vi "FMA1600A Add Units.vi"(0 "Meter Bank 2":T1, 1 "Meter Bank 1":T1, 5 "Meter Bank 3":T1, 7 "Measurement Units 1":T3, 9 "Measurement Units 2":T3, 12 "Measurement Units 3":T3) -> (2 "Display Bank 3":T1, 3 "Display S3":T4, 4 "Display Bank 2":T1, 6 "Display S2":T4, 8 "Display Bank 1":T1, 10 "Display S1":T4)   [LabVIEW 2016]
uses:
  Trunk/Range/Type Definitions/RANGE Panel Data.ctl
  Type Definitions/FMA1600A Gas Type.ctl
  Type Definitions/FMA1600A Units String.ctl
panel:
  out "Array":string[](array[string])
  out "Numeric":i32
  out "Error Out":errorcluster
  in  "Error In":errorcluster
  out "Controls[]":refnum<vi>[](array[refnum])
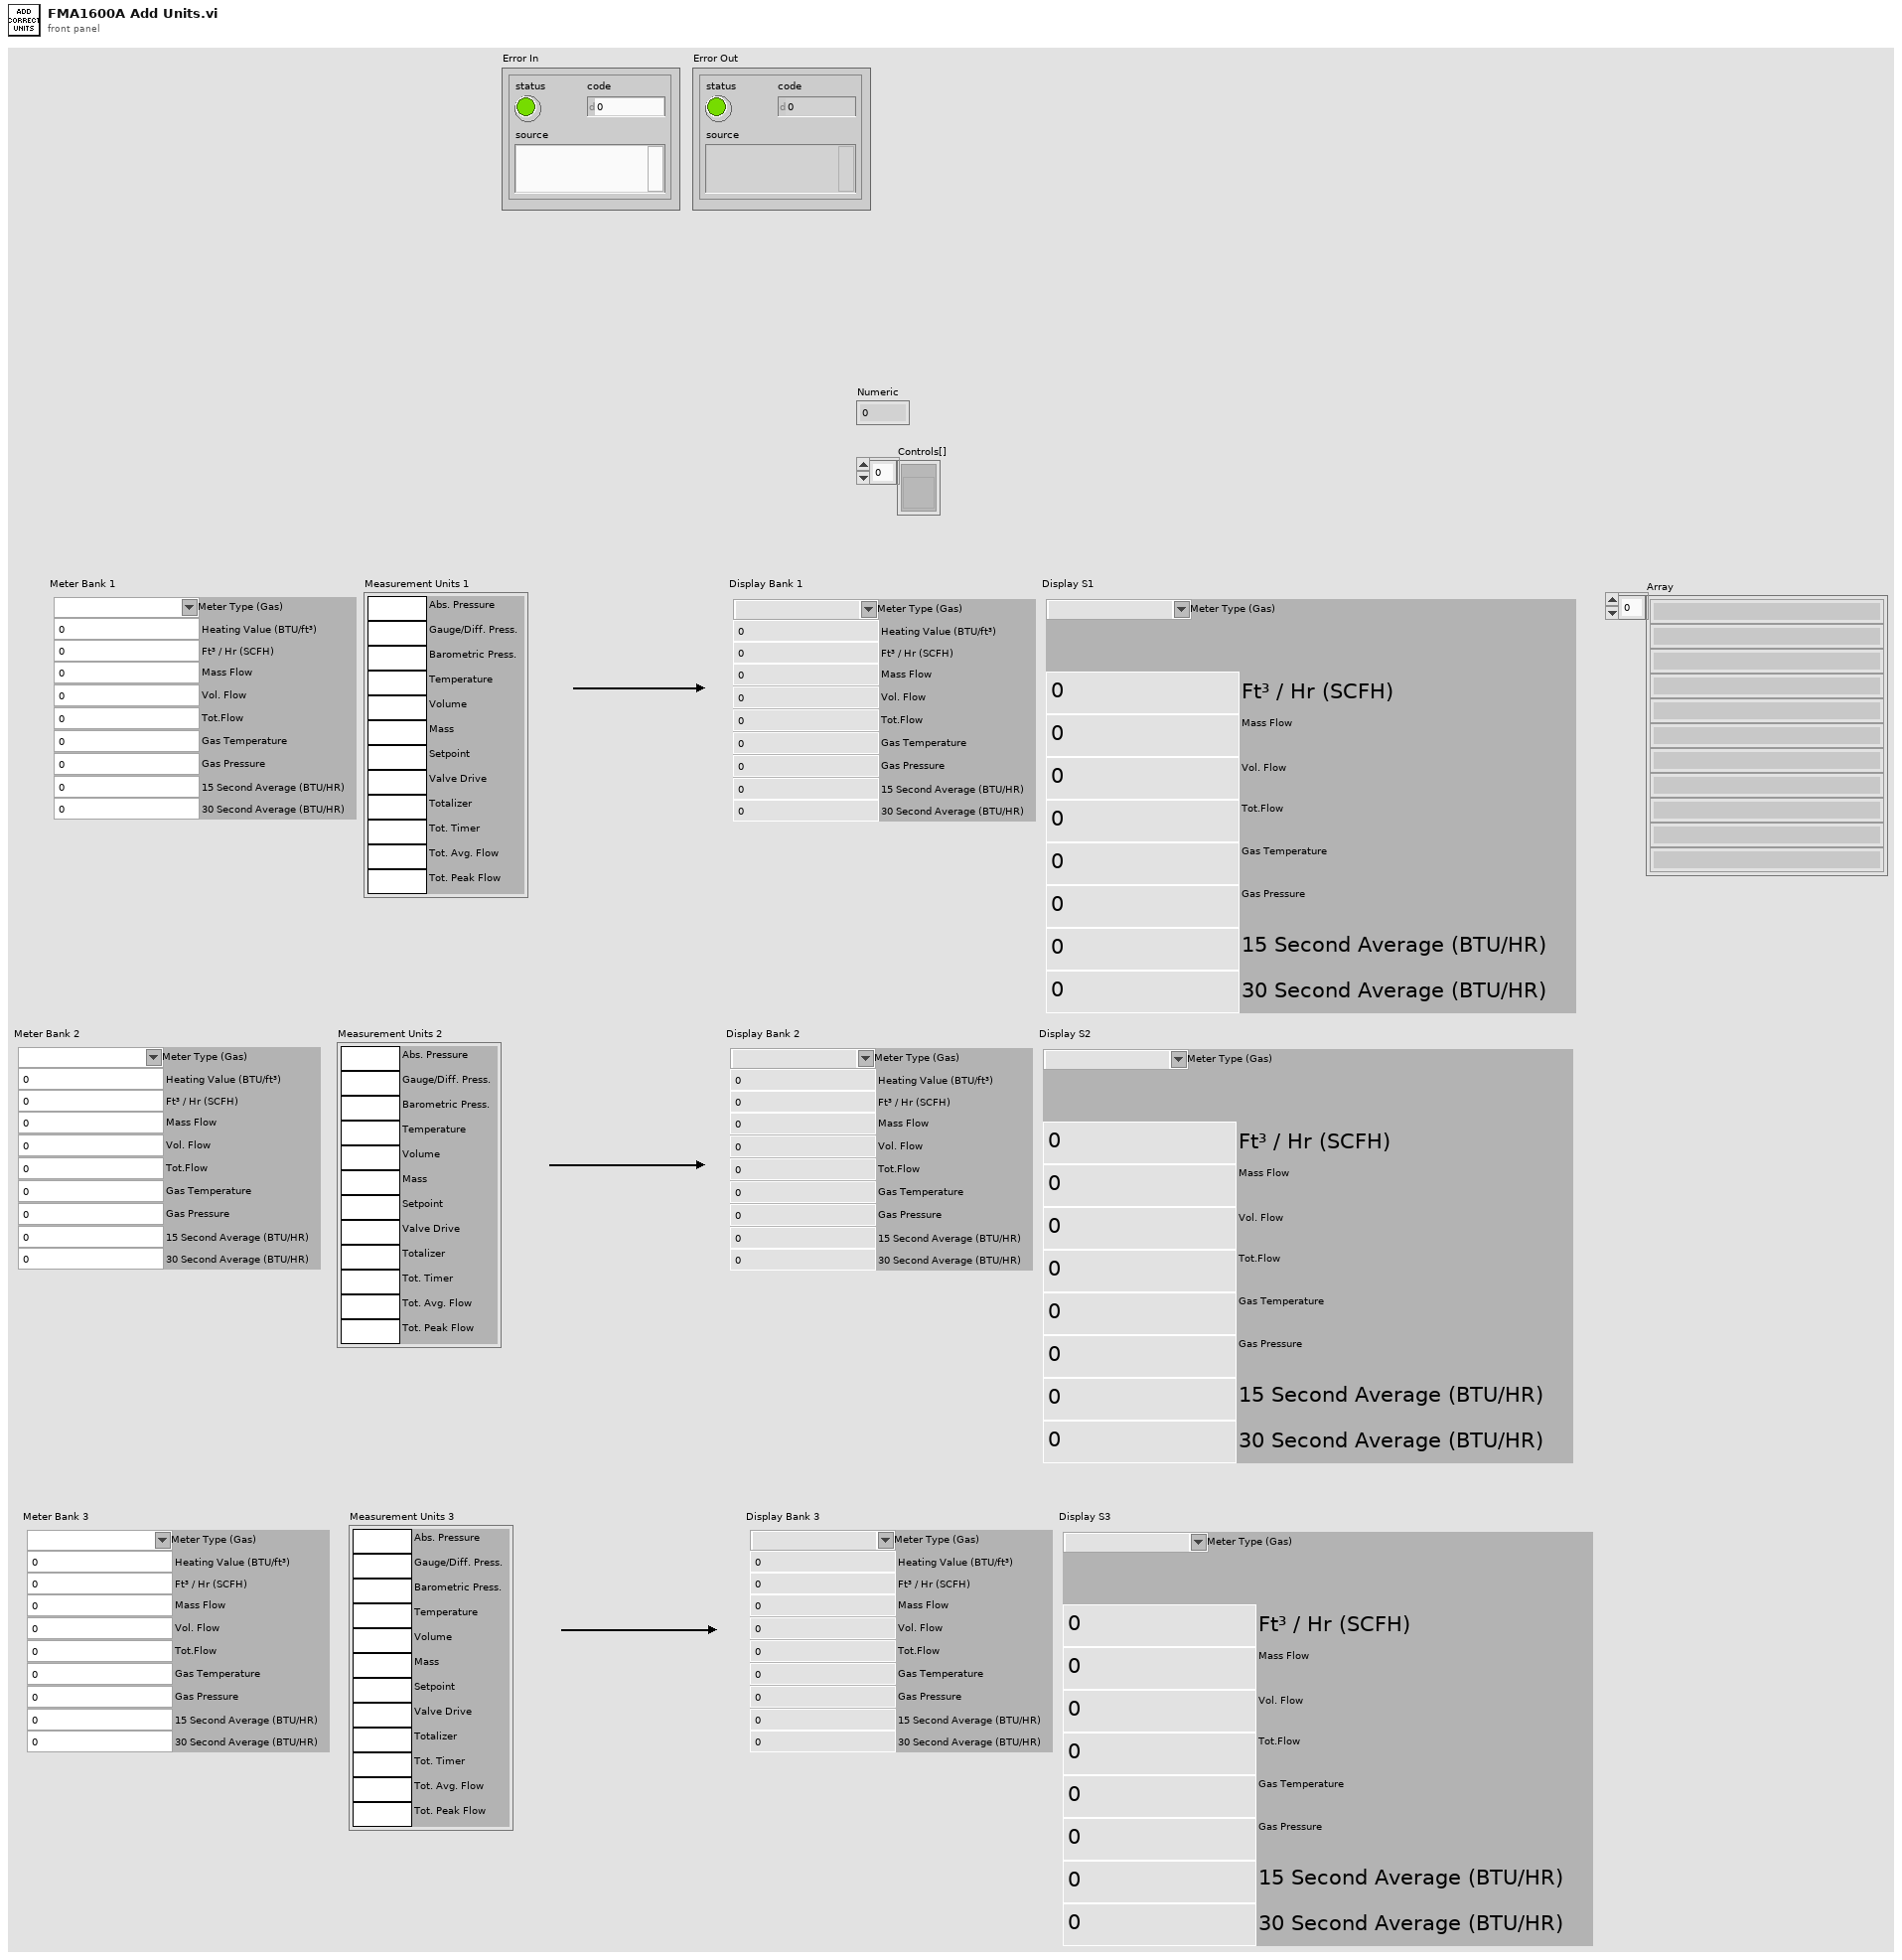
[diagram p1: front panel]
types:
  T1 = typedef "RANGE Panel Data.ctl" = cluster{"Meter Type (Gas)":T2, "Heating Value (BTU/ft³)":dbl, "Ft³ / Hr (SCFH)":dbl, "15 Second Average (BTU/HR)":dbl, "30 Second Average (BTU/HR)":dbl, "Mass Flow":dbl, "Vol. Flow":dbl, "Gas Temperature":dbl, "Gas Pressure":dbl, "Tot.Flow":dbl}
  T2 = typedef "FMA1600A Gas Type.ctl" = string
  T3 = typedef "FMA1600A Units String.ctl" = cluster{"Abs. Pressure":string, "Gauge/Diff. Press.":string, "Barometric Press.":string, "Temperature":string, "Volume":string, "Mass":string, "Setpoint":string, "Valve Drive":string, "Totalizer":string, "Tot. Timer":string, "Tot. Avg. Flow":string, "Tot. Peak Flow":string}
  T4 = cluster{"Meter Type (Gas)":T2, "Heating Value (BTU/ft³)":dbl, "Ft³ / Hr (SCFH)":dbl, "15 Second Average (BTU/HR)":dbl, "30 Second Average (BTU/HR)":dbl, "Mass Flow":dbl, "Vol. Flow":dbl, "Gas Temperature":dbl, "Gas Pressure":dbl, "Tot.Flow":dbl}
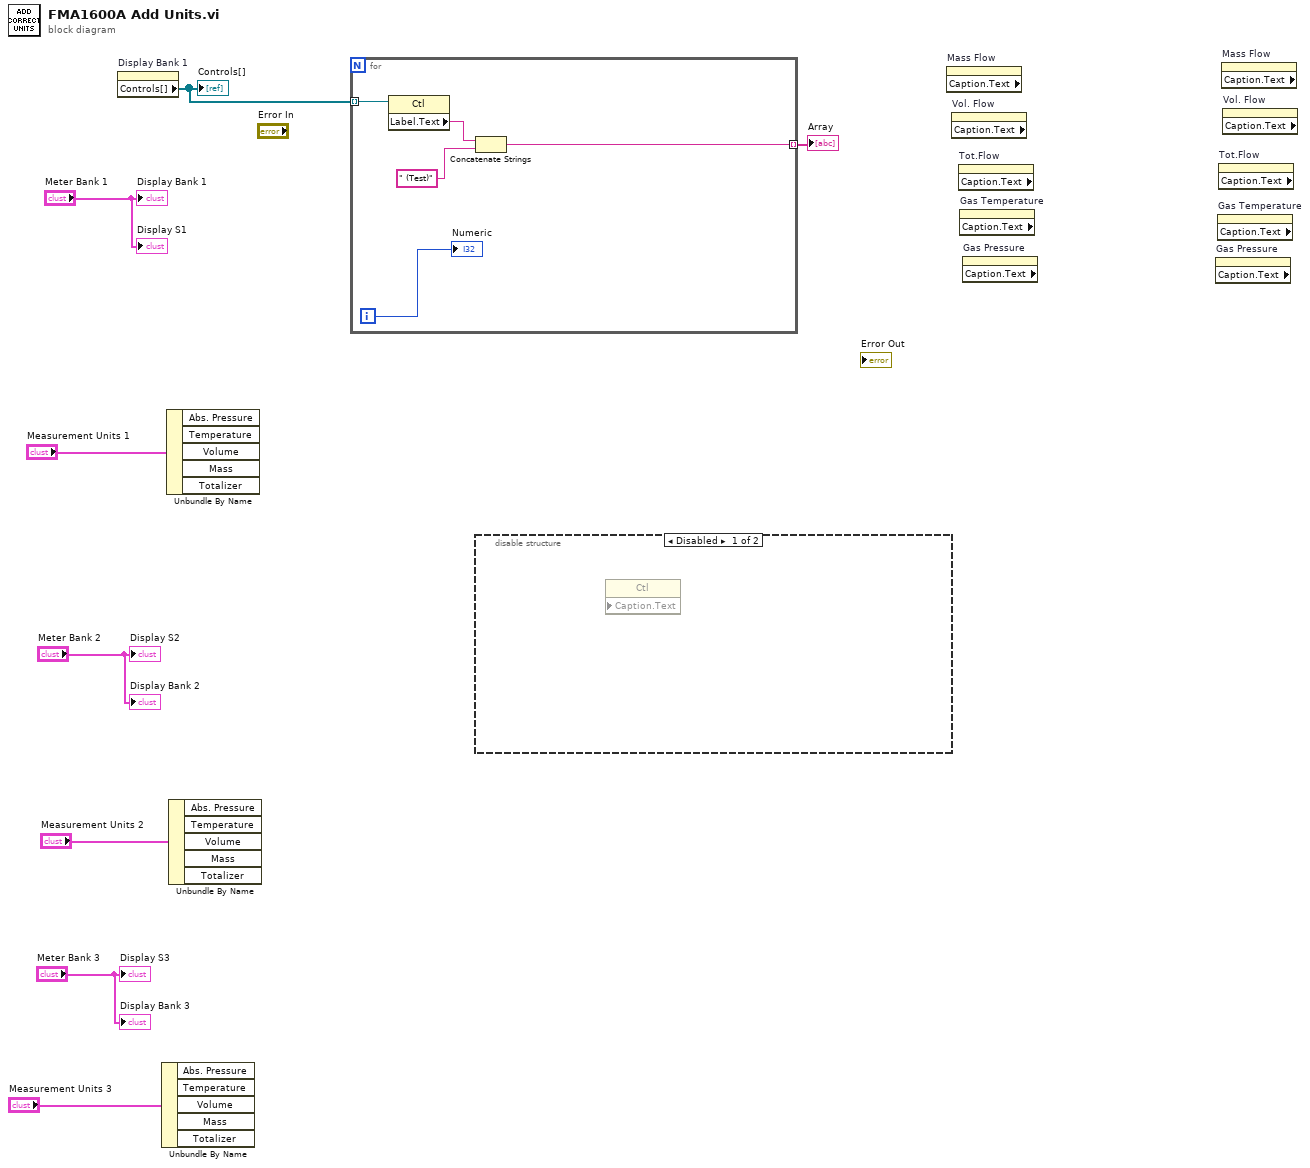
[diagram p0: block diagram]
diagram:
  n1 = property on="Display Bank 1" class="Clust (strict)"() -> ("Controls[]"=w2:refnum<vi>[])  [unwired: 2 in, 2 out]
  "Controls[]" <- w2
  n2 = Unbundle By Name("Measurement Units 3") -> ()  [unwired: 5 out]
  n3 = Unbundle By Name("Measurement Units 1") -> ()  [unwired: 5 out]
  n4 = Unbundle By Name("Measurement Units 2") -> ()  [unwired: 5 out]
  n5 = for {
    tunnel: w2 -> [w13] mode=indexing
    tunnel: [w9] -> w1 mode=indexing
    i -> [w10]
    n6 = property class="Ctl"(reference=w13) -> ("Label.Text"=w12:string)  [unwired: 1 in, 2 out]
    n7 = Concatenate Strings(w12, " (Test)") -> (w9:string)
    "Numeric" <- w10
  }
  "Array" <- w1
  n8 = disable-structure shown="Disabled" {
    frame Disabled {
      n9 = property class="Ctl" props=["Caption", "Text"]() -> ()  [unwired: 3 in, 2 out]
    }
    frame Enabled {
    }
  }
  n10 = property on="Mass Flow" class="DigNum (strict)" props=["Caption", "Text"]() -> ()  [unwired: 2 in, 3 out]
  n11 = property on="Vol. Flow" class="DigNum (strict)" props=["Caption", "Text"]() -> ()  [unwired: 2 in, 3 out]
  n12 = property on="Tot.Flow" class="DigNum (strict)" props=["Caption", "Text"]() -> ()  [unwired: 2 in, 3 out]
  n13 = property on="Gas Temperature" class="DigNum (strict)" props=["Caption", "Text"]() -> ()  [unwired: 2 in, 3 out]
  n14 = property on="Gas Pressure" class="DigNum (strict)" props=["Caption", "Text"]() -> ()  [unwired: 2 in, 3 out]
  n15 = property on="Gas Pressure" class="DigNum (strict)" props=["Caption", "Text"]() -> ()  [unwired: 2 in, 3 out]
  n16 = property on="Gas Temperature" class="DigNum (strict)" props=["Caption", "Text"]() -> ()  [unwired: 2 in, 3 out]
  n17 = property on="Tot.Flow" class="DigNum (strict)" props=["Caption", "Text"]() -> ()  [unwired: 2 in, 3 out]
  n18 = property on="Mass Flow" class="DigNum (strict)" props=["Caption", "Text"]() -> ()  [unwired: 2 in, 3 out]
  n19 = property on="Vol. Flow" class="DigNum (strict)" props=["Caption", "Text"]() -> ()  [unwired: 2 in, 3 out]
  "Display Bank 1" <- "Meter Bank 1"
  "Display Bank 2" <- "Meter Bank 2"
  "Display S1" <- "Meter Bank 1"
  "Display S2" <- "Meter Bank 2"
  "Display S3" <- "Meter Bank 3"
  "Display Bank 3" <- "Meter Bank 3"
